vi "Measure Single Point With Compliance.vi"(8 "error in (no error)":errorcluster, 11 "DMM_Base in":refnum<class "DMM_Base.lvclass">) -> (0 "error out":errorcluster, 1 "Out_Of_Range":bool, 2 "Measured_Value":dbl, 3 "DMM_Base out":refnum<class "DMM_Base.lvclass">)   [LabVIEW 2021, in "DMM_Base.lvclass"]
doc: "The API reads the single point measurement result for the given <b>Pin</b> along with Measurement Value Out of Range."
uses:
  DMM_Base.lvclass
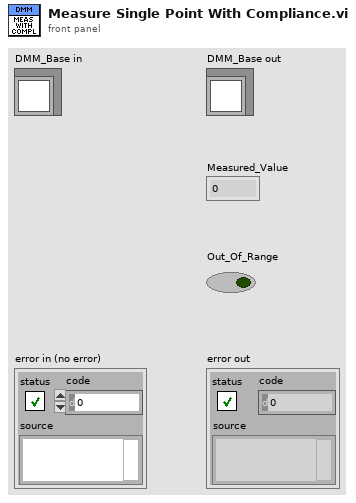
[diagram p1: front panel]
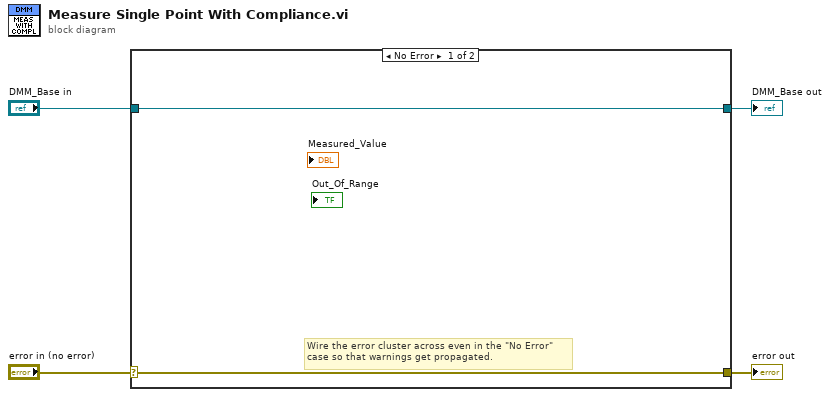
[diagram p0: block diagram]
diagram:
  n1 = case shown="No Error" "error in (no error)" {
    selector: "error in (no error)" -> [w5 w8]
    tunnel: [w5 w8] -> w3
    tunnel: [w6 w7] -> w1
    tunnel: "DMM_Base in" -> [w6 w7]
    frame No Error {
      # "Wire the error cluster across even in the \"No Error\"\ncase so that warnings get propagated."
    }
    frame Error {
    }
  }
  "error out" <- w3
  "DMM_Base out" <- w1
